vi "WPI_IMU_ADIS16448_AHRS_RoboBees.vi"(8 "Yaw Axis":enum16{"X", "Y", "Z"}(ring)=enum."Z", 10 "IMU Rates":dbl[](array[numeric])) -> (0 "Yaw":dbl(knob) scale=-180.0..180.0, 1 "Roll":dbl(knob) scale=-180.0..180.0, 2 "Pitch":dbl(knob) scale=-90.0..90.0, 3 "Output":cluster{"Pitch":dbl, "Roll":dbl, "Yaw":dbl})   [LabVIEW 2016, in "Apple Pi Gyro Library.lvlib" / "FRC_ADIS16448_IMU.lvlib"]
uses:
  FRC_ADIS16448_IMU.lvlib
panel:
  in  "Tilt Comp (Yaw)":bool=TRUE
  in  "tau mag":dbl=0.04
  in  "tau acc":dbl=0.95
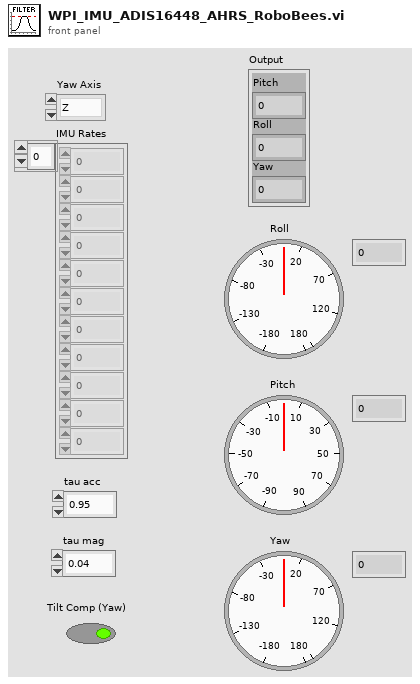
[diagram p1: front panel]
types:
  T1 = cluster{"Xaccel":dbl, "Yaccel":dbl, "Zaccel":dbl}
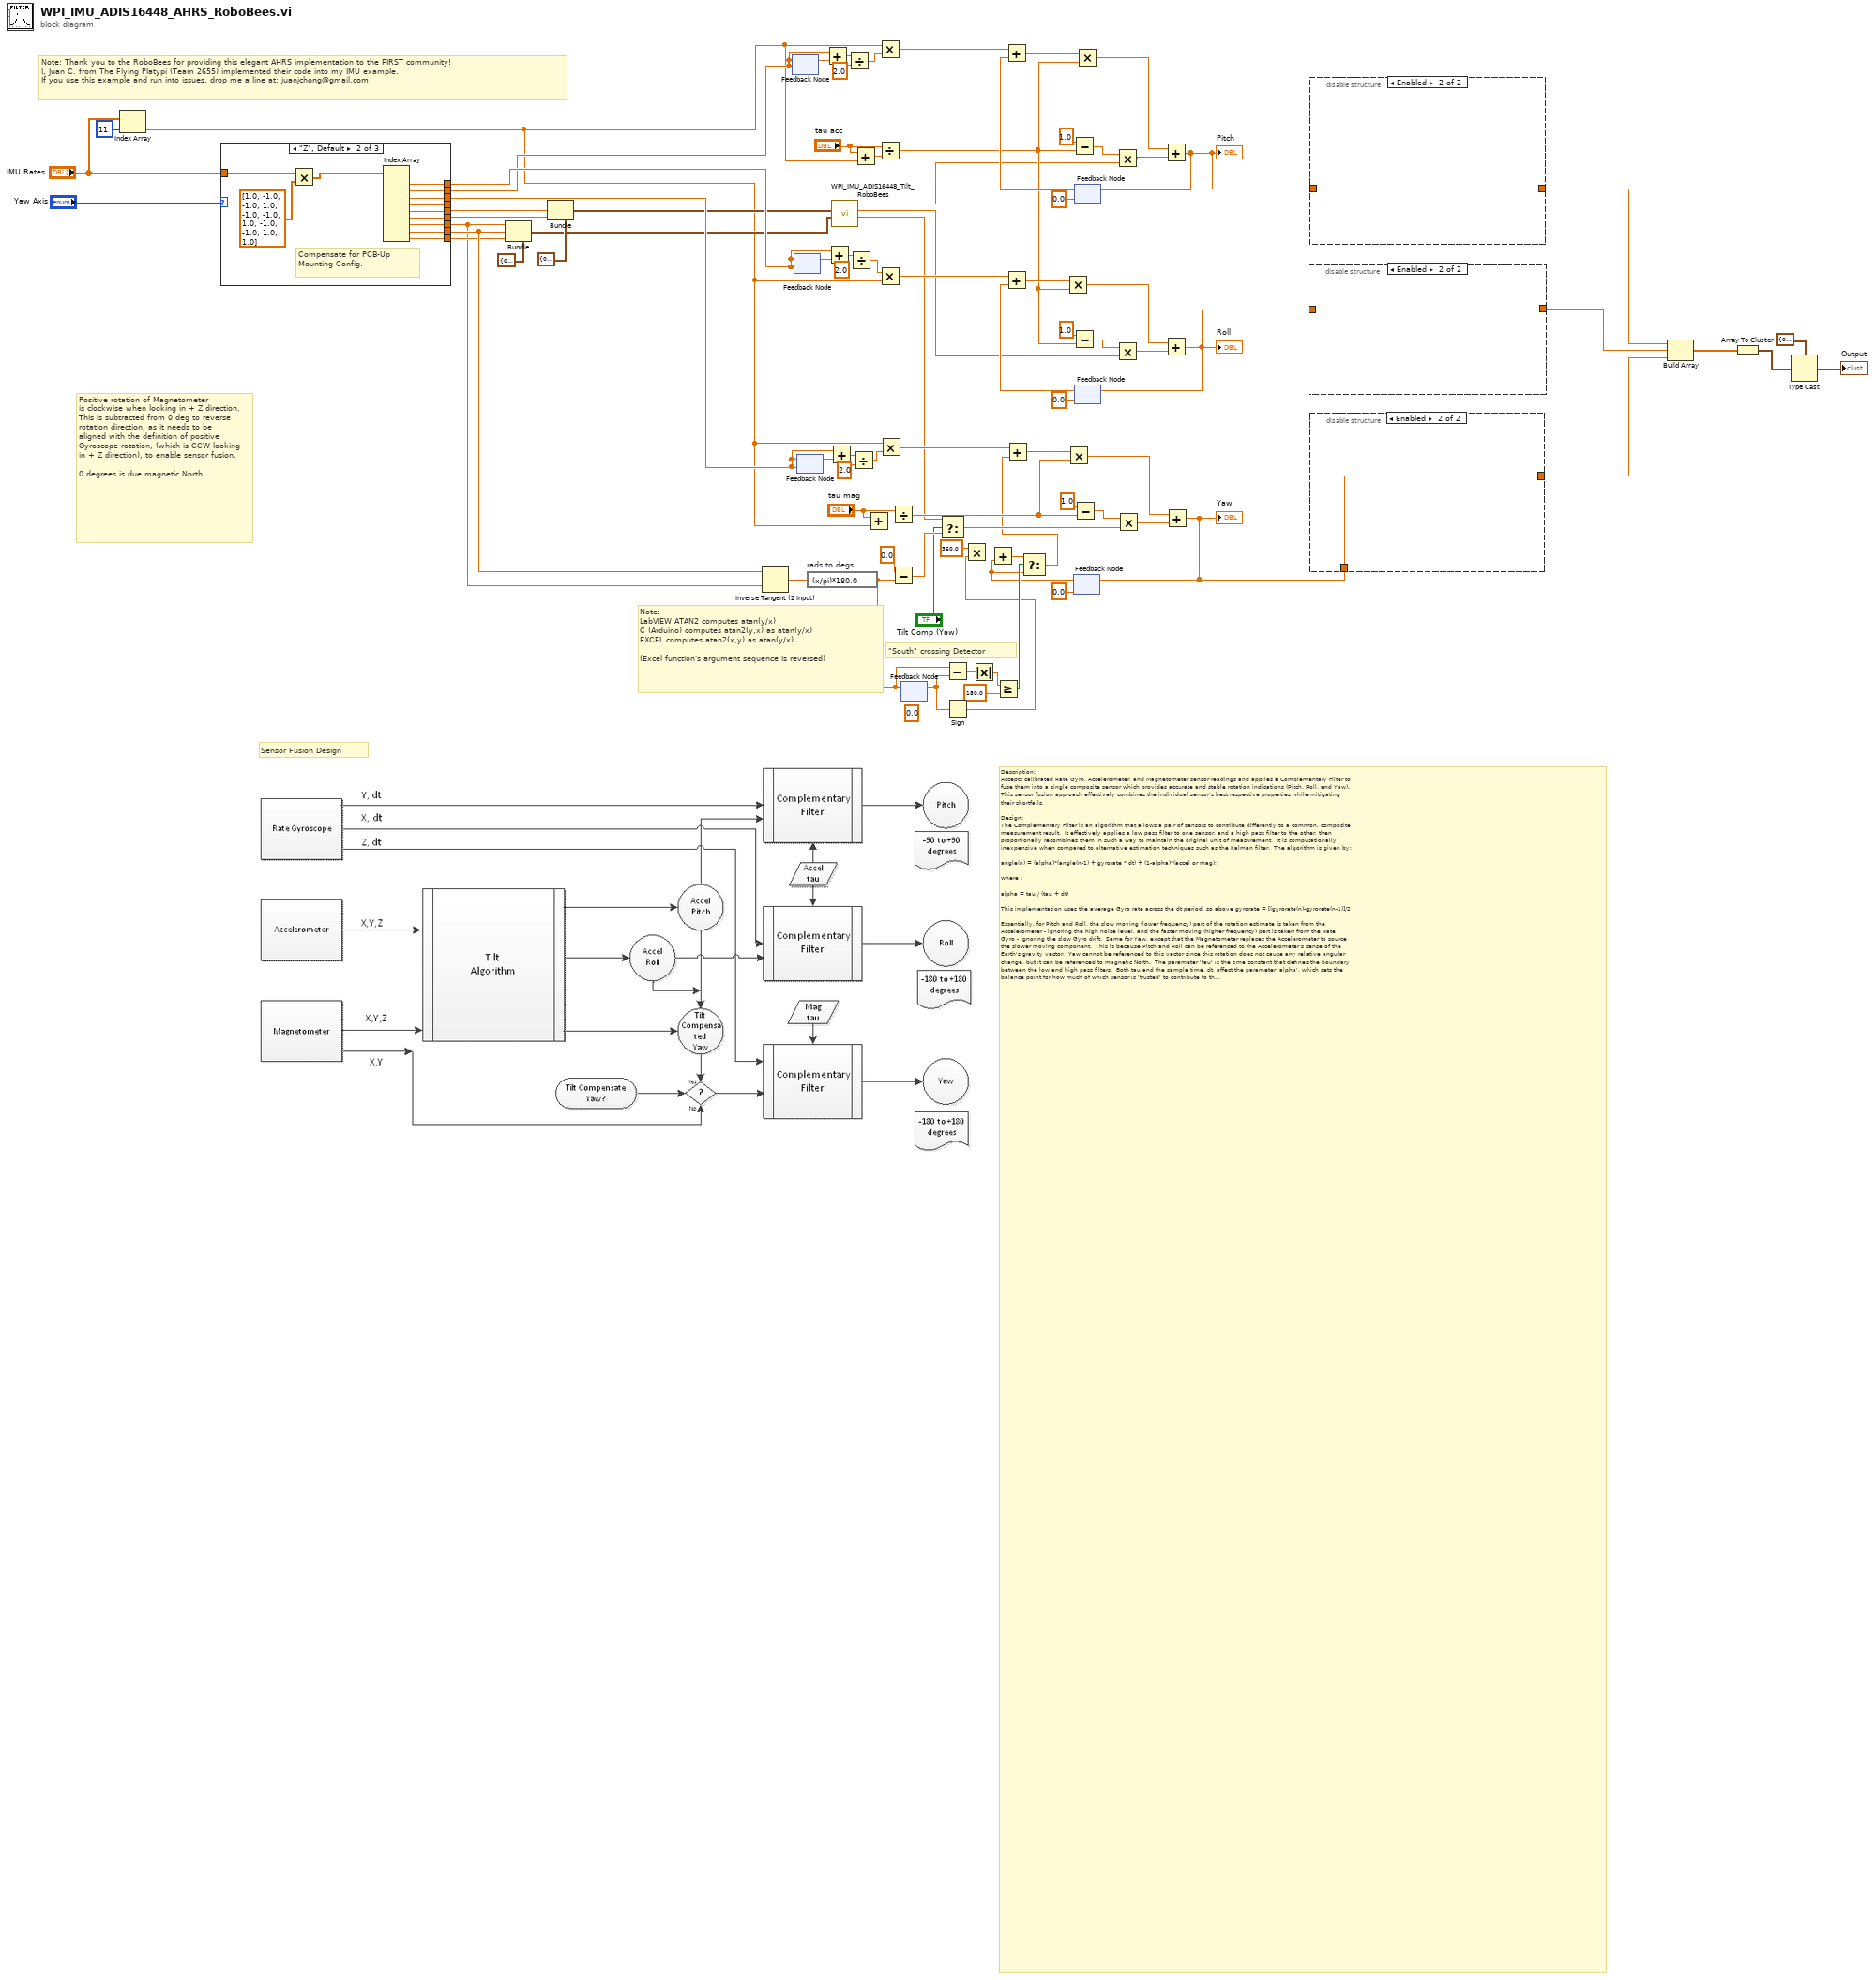
[diagram p0: block diagram]
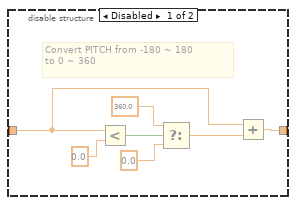
[diagram p2: hidden frame]
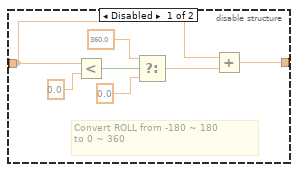
[diagram p3: hidden frame]
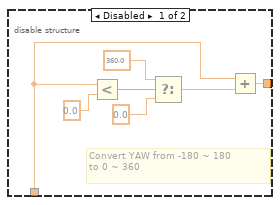
[diagram p4: hidden frame]
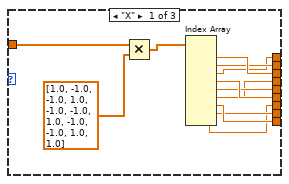
[diagram p5: hidden frame]
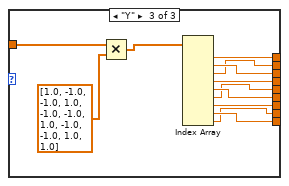
[diagram p6: hidden frame]
diagram:
  # "Note: Thank you to the RoboBees for providing this elegant AHRS implementation to the FIRST community!\nI, Juan C. from The Flying Platypi (Team 2655) implemented their code into my IMU example.\nIf you use this example and run into issues, drop me a line at: juanjchong@gmail.com"
  # "Sensor Fusion Design"
  # "Description:\nAccepts calibrated Rate Gyro, Accelerometer, and Magnetometer sensor readings and applies a Complementary Filter to\nfuse them into a single composite sensor which provides accurate and stable rotation indications (Pitch, Roll, and Yaw).\nThis sensor fusion approach effectively combines the individual sensor's best respective properties while mitigating\ntheir shortfalls.\n\nDesign:\nThe Complementary Filter is an algorithm that allows a pair of sensors to contribute differently to a common, composite\nmeasurement result.  It effectively applies a low pass filter to one sensor, and a high pass filter to the other, then\nproportionally recombines them in such a way to maintain the original unit of measurement.  It is computationally\ninexpensive when compared to alternative estimation techniques such as the Kalman filter.  The algorithm is given by:\n\nangle(n) = (alpha)*(angle(n-1) + gyrorate * dt) + (1-alpha)*(accel or mag);\n\nwhere : \n\nalpha = tau / (tau + dt)\n\nThis implementation uses the average Gyro rate across the dt period, so above gyrorate = [(gyrorate(n)-gyrorate(n-1)]/2\n\nEssentially, for Pitch and Roll, the slow moving (lower frequency) part of the rotation estimate is taken from the\nAccelerometer - ignoring the high noise level, and the faster moving (higher frequency) part is taken from the Rate \nGyro - ignoring the slow Gyro drift.  Same for Yaw, except that the Magnetometer replaces the Accelerometer to source\nthe slower moving component.  This is because Pitch and Roll can be referenced to the Accelerometer's sense of the\nEarth's gravity vector.  Yaw cannot be referenced to this vector since this rotation does not cause any relative angular\nchange, but it can be referenced to magnetic North.  The parameter 'tau' is the time constant that defines the boundary\nbetween the low and high pass filters.  Both tau and the sample time, dt, affect the parameter 'alpha', which sets the\nbalance point for how much of which sensor is 'trusted' to contribute to the rotation estimate.\n\nThe Complementary Filter algorithm is applied to each X/Y/Z rotation axis to compute R/P/Y outputs, respectively.\n\nMagnetometer readings are tilt-compensated when Tilt-Comp-(Yaw) is asserted (True), by the IMU TILT subVI.  This\ncreates what is known as a tilt-compensated compass, which allows Yaw to be insensitive to the effects of a\nnon-level sensor, but generates error in Yaw during movement (coordinate acceleration).\n\nThe Yaw \"South\" crossing detector is necessary to allow a smooth transition across the +/- 180 deg discontinuity (inherent\nin the ATAN function).  Since -180 deg is congruent with +180 deg, Yaw needs to jump between these values when\ncrossing South (North is 0 deg).  The design depends upon comparison of successive Yaw readings to detect a cross-over\nevent.  The cross-over detector monitors the current reading and evaluates how far it is from the previous reading.  If it\nis greater than the previous reading by the Discriminant (= 180 deg), then Yaw just crossed South.\n\nBy choosing 180 as the Discriminant, the only way the detector can produce a false positive, assuming a loop iteration\nof 70 msec, is for it to rotate >2,571 dps ... (2,571=180/.07).  This is faster than the ST L3GD20 Gyro can register.  The\ndetector produces a Boolean True upon detecting a South crossing.  This is used to alter the (n-1) Yaw which was\npreviously stored, either adding or subtracting 360 degrees as required to place the previous Yaw in the correct quadrant\nwhenever crossing occurs.  The Modulus function cannot be used here as the Complementary Filter algorithm has 'state'\n(needs to remember previous Yaw).\n \nWe are in effect stitching together two ends of a ruler for 'modular arithmetic' (clock math).\n\nInputs:\nGYRO - Gyro rate and sample time measurements.\nACCEL - Acceleration measurements.\nMAG - Magnetic measurements.\nTAU ACC - tau parameter used to set sensor balance between Accel and Gyro for Roll and Pitch.\nTAU MAG -  tau parameter used to set sensor balance between Mag and Gyro for Yaw.\nTILT COMP (Yaw) - Enables Yaw tilt-compensation if True.\n\nOutputs:\nROLL - Filtered Roll about sensor X-axis.\nPITCH - Filtered Pitch about sensor Y-axis.\nYAW - Filtered Yaw about sensor Z-axis.\n\nVI Properties:\nExecution Reentrancy is set to Non Reentrant Execution\n\nImplementation:\nIt's best to establish the optimum loop sample time first.  See IMU READ implementation notes for guidance.  Each\ntau parameter should then be adjusted to achieve optimum sensor fusion.  tau acc affects Roll and Pitch, tau mag affects\nYaw.  Start at value 1 or 2 and decrease by half each time until the result doesn't drift, but not so far that the result gets\nnoisy.  An optimum tau for this IMU is likely in the range of 1.0 to 0.01, for a loop sample time between 10 and 100 ms.\n\nNote that both sample timing (dt) and tau both affect the balance parameter, 'alpha'.  Adjusting either dt or tau will\nrequire the other to be readjusted to maintain a particular filter performance.\n\nIt is likely best to set Yaw tilt-compensation to off (False) if the Yaw value is to be used as feedback in a closed loop\ncontrol application.  The tradeoff is that Yaw will only be accurate while the robot is level.\n\nSince a Yaw of -180 degrees is congruent with +180 degrees (they represent the same direction), it is possible that the\nYaw output will oscillate between these two values when the sensor happens to be pointing due South, as sensor\nnoise causes slight variation.  You will need to account for this possibility if you are using the Yaw value for decision-\nmaking in code.\n\n----- The RoboBees FRC Team 836! -----  Complement your passion to solve problems with a STEM Education!"
  # "\"South\" crossing Detector"
  # "Positive rotation of Magnetometer\nis clockwise when looking in + Z direction.  This is subtracted from 0 deg to reverse rotation direction, as it needs to be aligned with the definition of positive Gyroscope rotation, (which is CCW looking in + Z direction), to enable sensor fusion.\n\n0 degrees is due magnetic North."
  # "Note:\nLabVIEW ATAN2 computes atan(y/x)\nC (Arduino) computes atan2(y,x) as atan(y/x)\nEXCEL computes atan2(x,y) as atan(y/x)\n\n(Excel function's argument sequence is reversed)"
  n1 = Index Array(array="IMU Rates", index=11) -> (element=w7:dbl)
  n2 = case shown="\"Z\", Default" "Yaw Axis" {
    tunnel: [w99 w113 w125] -> w29
    tunnel: [w96 w112 w122] -> w22
    tunnel: "IMU Rates" -> [w92 w104 w116]
    tunnel: [w93 w111 w119] -> w24
    tunnel: [w97 w110 w120] -> w21
    tunnel: [w98 w109 w121] -> w20
    tunnel: [w100 w108 w123] -> w28
    tunnel: [w101 w107 w124] -> w27
    tunnel: [w94 w106 w117] -> w26
    tunnel: [w95 w105 w118] -> w25
    frame "X" {
      n3 = Multiply(x=w92, y=dbl[] [1.0, -1.0, -1.0, 1.0, -1.0, -1.0, 1.0, -1.0, -1.0, 1.0, 1.0]) -> (x*y=w91:dbl[])
      n4 = Index Array(array=w91) -> (element #1=w101:dbl, element #2=w100:dbl, element #3=w99:dbl, element #4=w98:dbl, element #5=w97:dbl, element #6=w96:dbl, element #7=w95:dbl, element #8=w94:dbl, element #9=w93:dbl)  [unwired: 9 in]
    }
    frame "Z", Default {
      # "Compensate for PCB-Up\nMounting Config."
      n5 = Multiply(x=w104, y=dbl[] [1.0, -1.0, -1.0, 1.0, -1.0, -1.0, 1.0, -1.0, -1.0, 1.0, 1.0]) -> (x*y=w102:dbl[])
      n6 = Index Array(array=w102) -> (element #1=w113:dbl, element #2=w108:dbl, element #3=w107:dbl, element #4=w112:dbl, element #5=w110:dbl, element #6=w109:dbl, element #7=w111:dbl, element #8=w106:dbl, element #9=w105:dbl)  [unwired: 9 in]
    }
    frame "Y" {
      n7 = Multiply(x=w116, y=dbl[] [1.0, -1.0, -1.0, 1.0, -1.0, -1.0, 1.0, -1.0, -1.0, 1.0, 1.0]) -> (x*y=w114:dbl[])
      n8 = Index Array(array=w114) -> (element #1=w125:dbl, element #2=w124:dbl, element #3=w123:dbl, element #4=w122:dbl, element #5=w121:dbl, element #6=w120:dbl, element #7=w119:dbl, element #8=w118:dbl, element #9=w117:dbl)  [unwired: 9 in]
    }
  }
  n9 = Bundle(cluster=cluster{"Xmag":dbl, "Ymag":dbl, "Zmag":dbl} {"Xmag"=0.0, "Ymag"=0.0, "Zmag"=0.0} ("Mag"), "Xmag"=w24, "Ymag"=w26, "Zmag"=w25) -> (w17:cluster{"Xmag":dbl, "Ymag":dbl, "Zmag":dbl})
  n10 = Bundle(cluster=T1 {"Xaccel"=0.0, "Yaccel"=0.0, "Zaccel"=0.0} ("Accel"), "Xaccel"=w22, "Yaccel"=w21, "Zaccel"=w20) -> (w18:T1)
  n11 = Inverse Tangent (2 Input)(1:w24, 2:w26) -> (0:w62:dbl)
  n12 = feedback #1(w28) -> (w51:dbl)
  n13 = feedback-in #1(w28) -> ()
  n14 = feedback #2(w29) -> (w45:dbl)
  n15 = feedback-in #2(w29) -> ()
  n16 = feedback #3(w27) -> (w43:dbl)
  n17 = feedback-in #3(w27) -> ()
  n18 = expression code="(x/pi)*180.0" "rads to degs"(w62) -> (w32:dbl)
  n19 = Add(x=w28, y=w51) -> (x+y=w50:dbl)
  n20 = Add(x=w29, y=w45) -> (x+y=w46:dbl)
  n21 = Add(x=w27, y=w43) -> (x+y=w42:dbl)
  n22 = call "WPI_IMU_ADIS16448_Tilt_RoboBees.vi"("Mag"=w17, "Accel"=w18) -> ("Yaw"=w14:dbl, "Roll"=w15:dbl, "Pitch"=w16:dbl)  [unwired: 6 in, 1 out]
  n23 = Divide(x=w50, y=2.0) -> (x/y=w48:dbl)
  n24 = Divide(x=w46, y=2.0) -> (x/y=w44:dbl)
  n25 = Divide(x=w42, y=2.0) -> (x/y=w40:dbl)
  n26 = Add(x="tau acc", y=w7) -> (x+y=w88:dbl)
  n27 = Add(x="tau mag", y=w7) -> (x+y=w63:dbl)
  n28 = Multiply(x=w7, y=w48) -> (x*y=w76:dbl)
  n29 = Divide(x="tau acc", y=w88) -> (x/y=w72:dbl)
  n30 = Multiply(x=w44, y=w7) -> (x*y=w86:dbl)
  n31 = Multiply(x=w7, y=w40) -> (x*y=w56:dbl)
  n32 = Divide(x="tau mag", y=w63) -> (x/y=w55:dbl)
  n33 = Subtract(x=0.0 ("y"), y=w32) -> (x-y=w59:dbl)
  n34 = feedback #4(0.0) -> (w33:dbl)
  n35 = feedback-in #4(w32) -> ()
  n36 = Select(t=w14, s="Tilt Comp (Yaw)", f=w59) -> (s? t:f=w60:dbl)
  n37 = Subtract(x=w32, y=w33) -> (x-y=w39:dbl)
  n38 = Sign(1:w33) -> (0:w35:dbl)
  n39 = Multiply(x=360.0 ("y"), y=w35) -> (x*y=w31:dbl)
  n40 = Absolute Value(x=w39) -> (abs(x)=w38:dbl)
  n41 = Greater Or Equal?(x=w38, y=180.0) -> (x >= y?=w36:bool)
  n42 = Subtract(x=1.0, y=w72) -> (x-y=w75:dbl)
  n43 = Subtract(x=1.0, y=w72) -> (x-y=w71:dbl)
  n44 = Subtract(x=1.0, y=w55) -> (x-y=w69:dbl)
  n45 = feedback #5(0.0) -> (w30:dbl)
  n46 = Add(x=w31, y=w30) -> (x+y=w52:dbl)
  n47 = Select(t=w52, s=w36, f=w30) -> (s? t:f=w53:dbl)
  n48 = Add(x=w56, y=w53) -> (x+y=w66:dbl)
  n49 = Multiply(x=w66, y=w55) -> (x*y=w68:dbl)
  n50 = feedback #6(0.0) -> (w80:dbl)
  n51 = Add(x=w76, y=w80) -> (x+y=w77:dbl)
  n52 = Multiply(x=w77, y=w72) -> (x*y=w79:dbl)
  n53 = feedback #7(0.0) -> (w70:dbl)
  n54 = Add(x=w86, y=w70) -> (x+y=w85:dbl)
  n55 = Multiply(x=w85, y=w72) -> (x*y=w83:dbl)
  n56 = Multiply(x=w75, y=w16) -> (x*y=w78:dbl)
  n57 = Multiply(x=w71, y=w15) -> (x*y=w84:dbl)
  n58 = Multiply(x=w69, y=w60) -> (x*y=w67:dbl)
  n59 = Add(x=w79, y=w78) -> (x+y=w2:dbl)
  "Pitch" <- w2
  n60 = feedback-in #6(w2) -> ()
  n61 = Add(x=w83, y=w84) -> (x+y=w1:dbl)
  "Roll" <- w1
  n62 = feedback-in #7(w1) -> ()
  n63 = Add(x=w68, y=w67) -> (x+y=w13:dbl)
  "Yaw" <- w13
  n64 = feedback-in #5(w13) -> ()
  n65 = disable-structure shown="Enabled" {
    disable-tunnel: w1 -> [w127 w133]
    disable-tunnel: [w126 w133] -> w11
    frame Disabled {
      # "Convert ROLL from -180 ~ 180 \nto 0 ~ 360"
      n66 = Less?(x=w127, y=0.0) -> (x < y?=w131:bool)
      n67 = Select(t=360.0, s=w131, f=0.0) -> (s? t:f=w128:dbl)
      n68 = Add(x=w127, y=w128) -> (x+y=w126:dbl)
    }
    frame Enabled {
    }
  }
  n69 = disable-structure shown="Enabled" {
    disable-tunnel: [w135 w141] -> w10
    disable-tunnel: w2 -> [w134 w141]
    frame Disabled {
      # "Convert PITCH from -180 ~ 180 \nto 0 ~ 360"
      n70 = Less?(x=w134, y=0.0) -> (x < y?=w139:bool)
      n71 = Select(t=360.0, s=w139, f=0.0) -> (s? t:f=w136:dbl)
      n72 = Add(x=w134, y=w136) -> (x+y=w135:dbl)
    }
    frame Enabled {
    }
  }
  n73 = disable-structure shown="Enabled" {
    disable-tunnel: w13 -> [w143 w149]
    disable-tunnel: [w142 w149] -> w12
    frame Disabled {
      # "Convert YAW from -180 ~ 180 \nto 0 ~ 360"
      n74 = Less?(x=w143, y=0.0) -> (x < y?=w147:bool)
      n75 = Select(t=360.0, s=w147, f=0.0) -> (s? t:f=w144:dbl)
      n76 = Add(x=w143, y=w144) -> (x+y=w142:dbl)
    }
    frame Enabled {
    }
  }
  n77 = Build Array(w10, w11, w12) -> (w4:dbl[])
  n78 = Array To Cluster(array=w4) -> (cluster=w5:cluster{"[0]":dbl, "[1]":dbl, "[2]":dbl})
  n79 = Type Cast(type=cluster{"Pitch":dbl, "Roll":dbl, "Yaw":dbl} {"Pitch"=0.0, "Roll"=0.0, "Yaw"=0.0} ("IMU AHRS"), x=w5) -> (*(type *) &x=→"Output":cluster{"Pitch":dbl, "Roll":dbl, "Yaw":dbl})
